vi "Panel by Type.vi"(10 "Type":T1) -> (2 "ColumnPanel":refnum<class "ColumnPanel.lvclass">)   [LabVIEW 2020, in "Conditum-Tools.lvlib" / "Entity Editor.lvclass"]
uses:
  Entity Editor.lvclass
  Conditum/Field Type.ctl
  ColumnPanel/ColumnPanel.lvclass
  BooleanPanel/BooleanPanel.lvclass
  C:/dev/lv20CE/lv-conditum/Conditum-Tools/ColumnPanel/ColumnPanel.lvclass
  IntegerPanel/IntegerPanel.lvclass
  DoublePanel/DoublePanel.lvclass
  TimestampPanel/TimestampPanel.lvclass
  StringPanel/StringPanel.lvclass
  TextPanel/TextPanel.lvclass
  RelationPanel/RelationPanel.lvclass
  Conditum/Conditum.lvlib
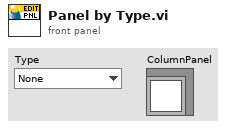
[diagram p1: front panel]
types:
  T1 = typedef "Conditum.lvlib/Field Type.ctl" = enum16{"None", "ID", "Boolean", "Integer", "Double", "Timestamp", "String", "Text", "Entity"}
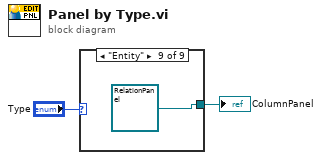
[diagram p0: block diagram]
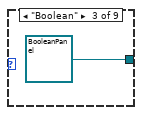
[diagram p4: hidden frame]
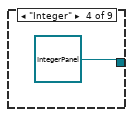
[diagram p5: hidden frame]
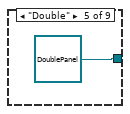
[diagram p6: hidden frame]
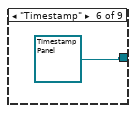
[diagram p7: hidden frame]
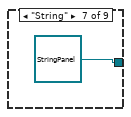
[diagram p8: hidden frame]
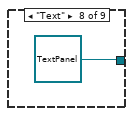
[diagram p9: hidden frame]
diagram:
  n1 = case shown="\"Entity\"" "Type" {
    tunnel: [_ _ refnum<class "BooleanPanel.lvclass"> refnum ("Conditum-Tools.lvlib:BooleanPanel.lvclass") refnum<class "IntegerPanel.lvclass"> refnum ("Conditum-Tools.lvlib:IntegerPanel.lvclass") refnum<class "DoublePanel.lvclass"> refnum ("Conditum-Tools.lvlib:DoublePanel.lvclass") refnum<class "TimestampPanel.lvclass"> refnum ("Conditum-Tools.lvlib:TimestampPanel.lvclass") refnum<class "StringPanel.lvclass"> refnum ("Conditum-Tools.lvlib:StringPanel.lvclass") refnum<class "TextPanel.lvclass"> refnum ("Conditum-Tools.lvlib:TextPanel.lvclass") refnum<class "RelationPanel.lvclass"> refnum ("Conditum-Tools.lvlib:RelationPanel.lvclass")] -> w1
    frame "None" {
    }
    frame "ID" {
    }
    frame "Boolean" {
    }
    frame "Integer" {
    }
    frame "Double" {
    }
    frame "Timestamp" {
    }
    frame "String" {
    }
    frame "Text" {
    }
    frame "Entity" {
    }
  }
  "ColumnPanel" <- w1
